vi "ManipChangeScoringPosition.vi"(3 "Instruction String":string) -> (0 "Error Out":errorcluster, 1 "Advance Trigger":bool)   [LabVIEW 2020]
doc: "This VI changes the robot's scoring position.\n\nParameters:\n1. state --> the robot's scoring position number"
uses:
  GlobalDriverStationData.vi
  SafeParser_Integer.vi
  GlobalDriverStationCommands.vi
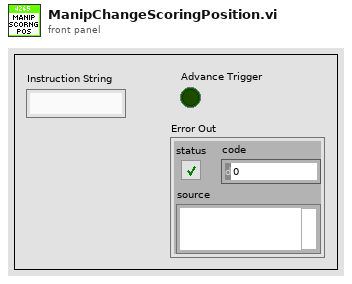
[diagram p1: front panel]
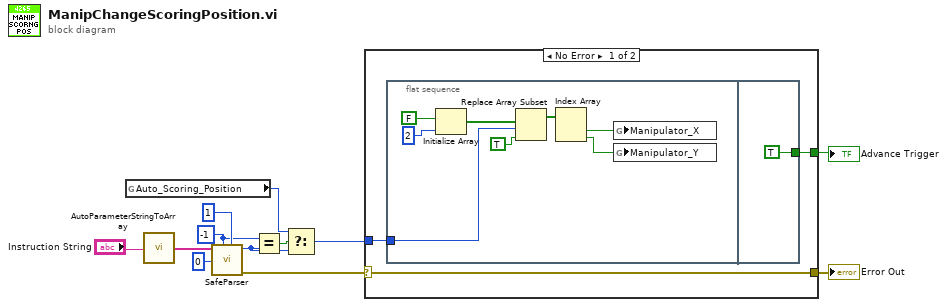
[diagram p0: block diagram]
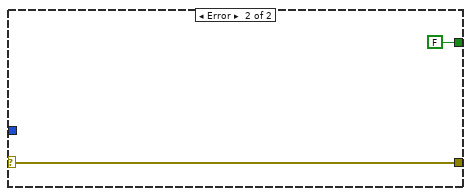
[diagram p2: hidden frame]
diagram:
  w5 = -1 ("Minimum")
  n1 = global read "GlobalDriverStationData.vi" "Auto_Scoring_Position"() -> (w2:i32)
  n2 = call "AutoParameterStringToArray.vi"("Parameter String"="Instruction String") -> ("Parsed Parameters"=w8:string[])
  n3 = call-poly "SafeParser.vi"("Maximum"=1, "Minimum"=w5, "Array Index"=0 ("Parameter Index"), "String Array"=w8) -> ("Error Out"=w10:errorcluster, "Typecast  Value"=w3:i32)  [unwired: 6 in]
  n4 = Equal?(x=w5, y=w3) -> (x = y?=w4:bool)
  n5 = Select(t=w2, s=w4, f=w3) -> (s? t:f=w1:i32)
  n6 = case shown="No Error" w10 {
    selector: w10 -> [w14 w26]
    tunnel: [w15 FALSE ("Advance Trigger")] -> w12
    tunnel: [w14 w26] -> w11
    tunnel: w1 -> [w13 _]
    frame No Error {
      n7 = flat-sequence {
        tunnel: w13 -> [w20]
        tunnel: [TRUE ("Advance Trigger")] -> w15
        frame #0 {
          n8 = Initialize Array(FALSE, 2 ("dimension size")) -> (w21:bool[])
          n9 = Replace Array Subset(array=w21, new element=TRUE ("new element/subarray"), index=w20) -> (w18:bool[])
          n10 = Index Array(array=w18) -> (element #1=w17:bool, element #2=w16:bool)  [unwired: 2 in]
          n11 = global write "GlobalDriverStationCommands.vi" "Manipulator_X"(w17) -> ()
          n12 = global write "GlobalDriverStationCommands.vi" "Manipulator_Y"(w16) -> ()
        }
        frame #1 {
        }
      }
    }
    frame Error {
    }
  }
  "Advance Trigger" <- w12
  "Error Out" <- w11
